vi "Add DTC.vi"(7 "DTC Type":enum8{"DM1 - Active", "DM2 - Previously Active"}(ring), 8 "error in (no error)":errorcluster, 10 "Name":string, 11 "Device Ref in":T1 format="%.0x") -> (0 "error out":errorcluster, 3 "Device Ref out":T1 format="%.0x")   [LabVIEW 2023, in "J1939 System Definition API Support.lvlib"]
uses:
  J1939 System Definition API Support.lvlib
  <vilib>/NI VeriStand/Custom Device API/Custom Device Item Ref.ctl
  Addon/Addon Shared/SubVIs/Constants.vi
  <vilib>/NI/NI VeriStand Advanced SysDef API/_SubVIs/SysDef.Search.GUID.vi
  Addon/Addon Shared/J1939 Addon Shared.lvlib
  <vilib>/NI/NI VeriStand Advanced SysDef API/SysDef API/Advanced System Definition.lvlib
  <vilib>/NI VeriStand/Custom Device API/Custom Device API.lvlib
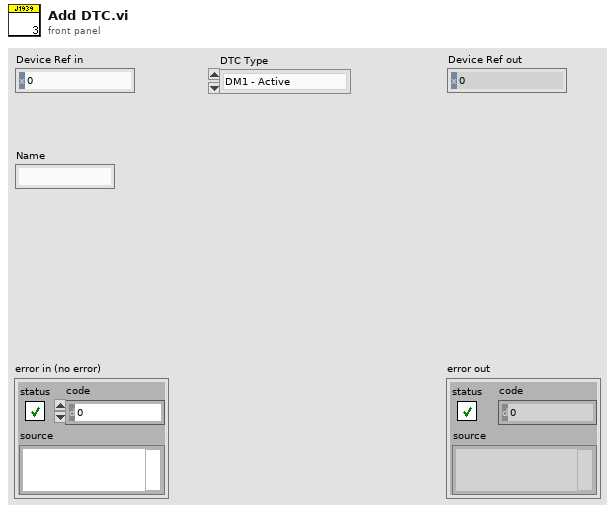
[diagram p1: front panel]
types:
  T1 = typedef "Custom Device API.lvlib/Custom Device Item Ref.ctl" = u64
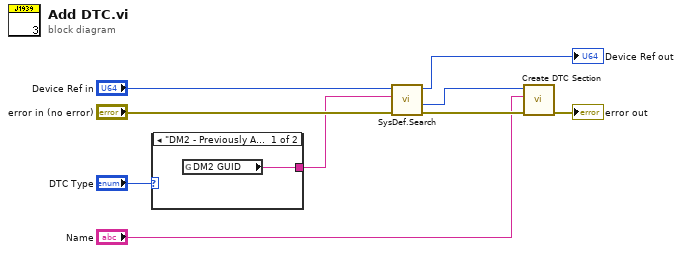
[diagram p0: block diagram]
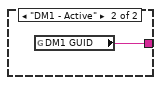
[diagram p2: hidden frame]
diagram:
  n1 = case shown="\"DM2 - Previously Active\"" "DTC Type" {
    tunnel: [w10 w11] -> w8
    frame "DM2 - Previously Active" {
      n2 = global read "Constants.vi" "DM2 GUID"() -> (w10:string)
    }
    frame "DM1 - Active" {
      n3 = global read "Constants.vi" "DM1 GUID"() -> (w11:string)
    }
  }
  n4 = call-poly <vilib>:"SysDef.Search.vi"("error in (no error)"="error in (no error)", "GUID"=w8, "nodeID"="Device Ref in") -> ("error out"=w4:errorcluster, "Value out"=w5:u64, "nodeID out"=→"Device Ref out":u64)  [unwired: 5 in, 1 out]
  n5 = call "Create DTC Section.vi"("error in (no error)"=w4, "Name"="Name", "Item Ref in"=w5) -> ("error out"=→"error out":errorcluster)  [unwired: 8 in]
